vi "Compuerta_Con.vi"(9 "FALLA":bool, 10 "CONSOLIDACION":bool, 11 "SATURACION":bool) -> (3 "Boolean":bool)   [LabVIEW 2013]
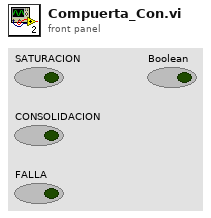
[diagram p1: front panel]
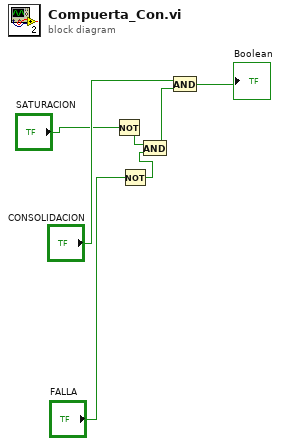
[diagram p0: block diagram]
diagram:
  n1 = Not(x="SATURACION") -> (.not. x?=w5:bool)
  n2 = Not(x="FALLA") -> (.not. x?=w4:bool)
  n3 = And(x=w5, y=w4) -> (x .and. y?=w6:bool)
  n4 = And(x="CONSOLIDACION", y=w6) -> (x .and. y?=→"Boolean":bool)
